vi "InsertArgs.vi"(10 "Arguments":T2, 11 "StepIn":T1) -> (3 "StepOut":T1)   [LabVIEW 2016]
uses:
  <vilib>/regexp/Match Regular Expression.xnode
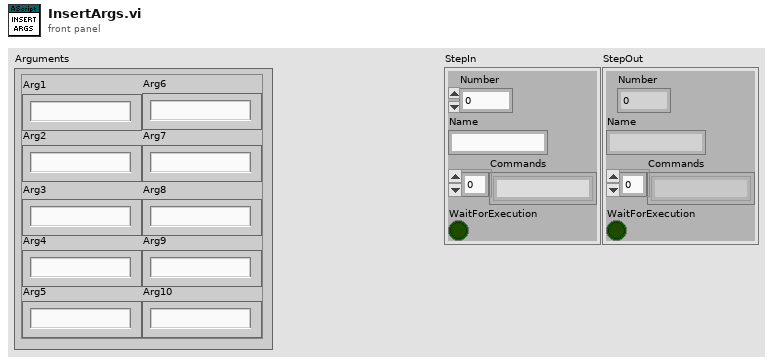
[diagram p1: front panel]
types:
  T1 = cluster{"Number":i32, "Name":string, "Commands":string[], "WaitForExecution":bool}
  T2 = cluster{"Arg1":string, "Arg2":string, "Arg3":string, "Arg4":string, "Arg5":string, "Arg6":string, "Arg7":string, "Arg8":string, "Arg9":string, "Arg10":string}
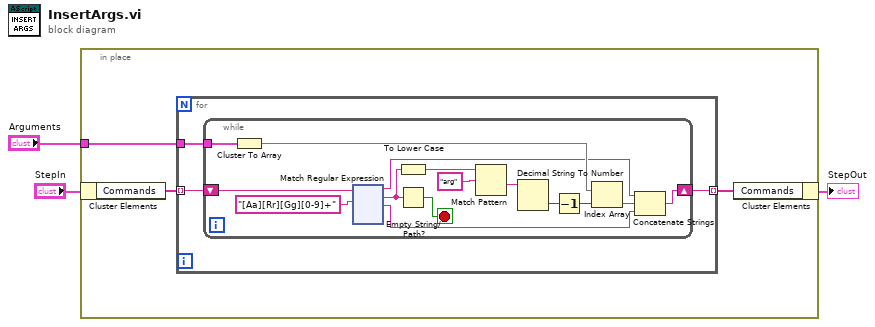
[diagram p0: block diagram]
diagram:
  n1 = in-place {
    in-place-border: "Arguments" -> [w6]
    n2 = in-place-cluster #1("StepIn") -> ("Commands"=w5:string[])
    n3 = for {
      tunnel: w5 -> [w9] mode=indexing
      tunnel: w6 -> [w8]
      tunnel: [w7] -> w4 mode=indexing
      n4 = while {
        shift-right: [w10] -> w7
        shift-left: w9 -> [w23]
        tunnel: w8 -> [w17]
        stop <- w22 stop-if-true
        n5 = Cluster To Array(cluster=w17) -> (array=w14:string[])
        n6 = xnode "Match Regular Expression"("input string"=w23, "regular expression"="[Aa][Rr][Gg][0-9]+") -> ("before match"=w12:string, "whole match"=w21:string, "after match"=w11:string)  [unwired: 4 in, 2 out]
        n7 = To Lower Case(string=w21) -> (all lower case string=w20:string)
        n8 = Empty String/Path?(string/path=w21) -> (empty?=w22:bool)
        n9 = Match Pattern(string=w20, regular expression="arg") -> (after substring=w18:string)  [unwired: 1 in, 3 out]
        n10 = Decimal String To Number(string=w18) -> (number=w16:i32)  [unwired: 2 in, 1 out]
        n11 = Decrement(x=w16) -> (x-1=w15:i32)
        n12 = Index Array(array=w14, index=w15) -> (element=w13:string)
        n13 = Concatenate Strings(w12, w13, w11) -> (w10:string)
      }
    }
    n14 = in-place-cluster #1("Commands"=w4) -> (→"StepOut":T1)
  }
